vi "Unregister PVs.vi"(8 "error in (no error)":errorcluster, 10 "Unregister Info":T1, 11 "CS++PVMonitor in":refnum<class "CS++PVMonitor.lvclass">) -> (0 "error out":errorcluster, 3 "CS++PVMonitor out":refnum<class "CS++PVMonitor.lvclass">)   [LabVIEW 2015, in "CS++PVMonitor.lvlib" / "CS++PVMonitor.lvclass"]
doc: "Unregister value change monitoring for process variables."
uses:
  CS++PVMonitor.lvclass
  <vilib>/ActorFramework/Message Enqueuer/Message Enqueuer.lvclass
  CS++PVMonitor.lvclass/CS++PVMonitor.ctl
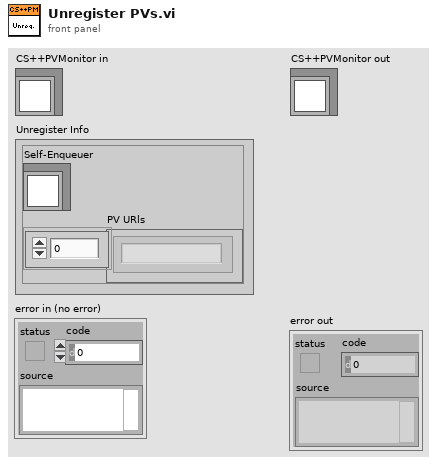
[diagram p1: front panel]
types:
  T1 = cluster{"Self-Enqueuer":refnum<class "Message Enqueuer.lvclass">, "PV URls":string[]}
  T2 = cluster{"PV URL":string, "Observers":cluster{"Enqueuer":refnum<class "Message Enqueuer.lvclass">, "CS++PVUpdate Msg":refnum<class "CS++PVUpdate Msg.lvclass">}[]}[]
  T3 = cluster{"PV URL":string, "Observers":cluster{"Enqueuer":refnum<class "Message Enqueuer.lvclass">, "CS++PVUpdate Msg":refnum<class "CS++PVUpdate Msg.lvclass">}[]}
  T4 = cluster{"Enqueuer":refnum<class "Message Enqueuer.lvclass">, "CS++PVUpdate Msg":refnum<class "CS++PVUpdate Msg.lvclass">}[]
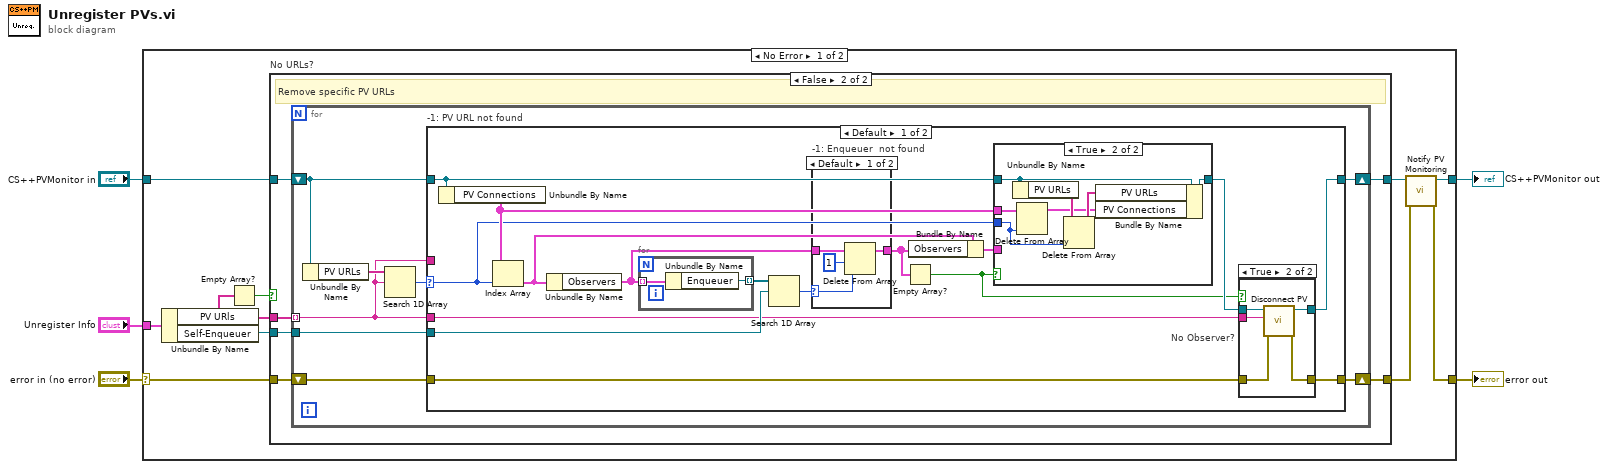
[diagram p0: block diagram]
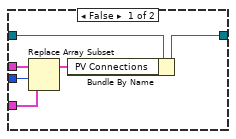
[diagram p3: hidden frame]
diagram:
  n1 = case shown="No Error" "error in (no error)" {
    selector: "error in (no error)" -> [w14 w78]
    tunnel: [w9 w78] -> w1
    tunnel: [w10 w77] -> w2
    tunnel: "CS++PVMonitor in" -> [w13 w77]
    tunnel: "Unregister Info" -> [w15 _]
    frame No Error {
      n2 = Unbundle By Name(w15) -> ("PV URls"=w7:string[], "Self-Enqueuer"=w12:refnum<class "Message Enqueuer.lvclass">)
      n3 = Empty Array?(array=w7) -> (empty?=w6:bool)
      n4 = case "No URLs?" shown="False" w6 {
        tunnel: w7 -> [_ w23]
        tunnel: w14 -> [w16 w22]
        tunnel: [w16 w21] -> w8
        tunnel: w13 -> [w17 w20]
        tunnel: [w17 w19] -> w11
        tunnel: w12 -> [_ w18]
        frame True {
          # "Remove observer from all PV URLs; to be implemented!"
        }
        frame False {
          # "Remove specific PV URLs"
          n5 = for {
            tunnel: w23 -> [w24] mode=indexing
            shift-right: [w26] -> w21
            shift-left: w22 -> [w25]
            shift-right: [w27] -> w19
            shift-left: w20 -> [w29]
            tunnel: w18 -> [w28]
            n6 = Unbundle By Name(w29) -> ("PV URLs"=w31:string[])
            n7 = Search 1D Array(1D array=w31, element=w24) -> (index of element=w30:i32)  [unwired: 1 in]
            n8 = case "-1: PV URL not found" shown="Default" w30 {
              selector: w30 -> [w44 _]
              tunnel: w29 -> [w35 w76]
              tunnel: w28 -> [w42 _]
              tunnel: w24 -> [w36 _]
              tunnel: [w39 w76] -> w27
              tunnel: [w37 w75] -> w26
              tunnel: w25 -> [w38 w75]
              tunnel: w24 -> [_ _]
              frame Default {
                n9 = Unbundle By Name(w35) -> ("PV Connections"=w45:T2)
                n10 = Index Array(array=w45, index=w44) -> (element=w43:T3)
                n11 = Unbundle By Name(w43) -> ("Observers"=w46:T4)
                n12 = for {
                  tunnel: w46 -> [w74] mode=indexing
                  tunnel: [w73] -> w47 mode=indexing
                  n13 = Unbundle By Name(w74) -> ("Enqueuer"=w73:refnum<class "Message Enqueuer.lvclass">)
                }
                n14 = Search 1D Array(1D array=w47, element=w42) -> (index of element=w40:i32)  [unwired: 1 in]
                n15 = case "-1: Enqueuer  not found" shown="Default" w40 {
                  selector: w40 -> [w69 _]
                  tunnel: w46 -> [w71 w72]
                  tunnel: [w70 w72] -> w32
                  frame Default {
                    n16 = Delete From Array(array=w71, length=1, index=w69) -> (array with subset deleted=w70:T4)  [unwired: 1 out]
                  }
                  frame -1 {
                  }
                }
                n17 = Empty Array?(array=w32) -> (empty?=w33:bool)
                n18 = Bundle By Name(cluster=w43, "Observers"=w32) -> (w41:T3)
                n19 = case shown="True" w33 {
                  tunnel: w45 -> [w53 w60]
                  tunnel: w44 -> [w52 w58]
                  tunnel: w41 -> [w51 _]
                  tunnel: w35 -> [w50 w57]
                  tunnel: [w49 w55] -> w34
                  frame False {
                    n20 = Replace Array Subset(array=w53, new element=w51, index=w52) -> (w48:T2)
                    n21 = Bundle By Name(cluster=w50, "PV Connections"=w48) -> (w49:refnum<class "CS++PVMonitor.lvclass">)
                  }
                  frame True {
                    n22 = Unbundle By Name(w57) -> ("PV URLs"=w59:string[])
                    n23 = Delete From Array(array=w60, index=w58) -> (array with subset deleted=w54:T2)  [unwired: 1 in, 1 out]
                    n24 = Delete From Array(array=w59, index=w58) -> (array with subset deleted=w56:string[])  [unwired: 1 in, 1 out]
                    n25 = Bundle By Name(cluster=w57, "PV URLs"=w56, "PV Connections"=w54) -> (w55:refnum<class "CS++PVMonitor.lvclass">)
                  }
                }
                n26 = case "No Observer?" shown="True" w33 {
                  tunnel: w34 -> [w62 w67]
                  tunnel: [w62 w66] -> w39
                  tunnel: w38 -> [w61 w65]
                  tunnel: [w61 w64] -> w37
                  tunnel: w36 -> [_ w63]
                  frame False {
                  }
                  frame True {
                    n27 = call-dynamic "Disconnect PV.vi"("error in (no error)"=w65, "PV URL"=w63, "CS++PVMonitor in"=w67) -> ("error out"=w64:errorcluster, "CS++PVMonitor out"=w66:refnum<class "CS++PVMonitor.lvclass">)  [unwired: 7 in]
                  }
                }
              }
              frame -1 {
              }
            }
          }
        }
      }
      n28 = call-dynamic "Notify PV Monitoring.vi"("error in (no error)"=w8, "CS++PVMonitor in"=w11) -> ("error out"=w9:errorcluster, "CS++PVMonitor out"=w10:refnum<class "CS++PVMonitor.lvclass">)  [unwired: 8 in]
    }
    frame Error {
    }
  }
  "error out" <- w1
  "CS++PVMonitor out" <- w2
